vi "periodicTasksRefNum.vi"() -> (1 "Refnums":T28)   [LabVIEW 2016]
uses:
  <vilib>/Rock Robotics/WPI/RobotDrive/WPI_RobotDriveDevRef.ctl
  <vilib>/Rock Robotics/WPI/MotorControl/WPI_MotorControlDeviceRef.ctl
  <vilib>/Rock Robotics/WPI/MotorControl/WPI_MotorControlType.ctl
  <vilib>/Rock Robotics/SystemInterfaces/DIO/FPGA_DIOPWMChannel.ctl
  <vilib>/Rock Robotics/WPI/PWM/WPI_PWMDeadband.ctl
  Sensors/PixyCam/Private/PixyCam_DevRef.ctl
  Sensors/PixyCam/Private/PixyCam_SPI_DevRef.ctl
  <vilib>/Rock Robotics/WPI/SPI/WPI_SPIDevRef.ctl
  <vilib>/Rock Robotics/SystemInterfaces/spilib/spi_bus.ctl
  Sensors/PixyCam/Private/PixyCam_CommMode.ctl
  Sensors/ADI MXP IMU/ADI_IMU_ADIS16448_InterruptDevRef.ctl
  Sensors/ADI MXP IMU/ADI_IMU_ADIS16448_IMUDevRef.ctl
  <vilib>/Rock Robotics/WPI/Interrupt/WPI_InterruptRef.ctl
  <vilib>/Rock Robotics/SystemInterfaces/Interrupt/FPGA_InterruptIndex.ctl
  <vilib>/Rock Robotics/WPI/AnalogChannel/WPI_AnalogChannelDevRef.ctl
  <vilib>/Rock Robotics/SystemInterfaces/AI/FPGA_AIChannel.ctl
  <vilib>/Rock Robotics/WPI/Ultrasonic/WPI_SonarMB1010DigitalDeviceRef.ctl
  <vilib>/Rock Robotics/WPI/Counter/WPI_CounterDevRef.ctl
  <vilib>/Rock Robotics/SystemInterfaces/Counter/FPGA_CounterCtrSystemIndex.ctl
  <vilib>/Rock Robotics/WPI/Encoder/WPI_EncoderDevRef.ctl
  <vilib>/Rock Robotics/SystemInterfaces/Encoder/FPGA_EncoderIdx.ctl
  <vilib>/Rock Robotics/WPI/Encoder/WPI_EncoderType.ctl
  <vilib>/Rock Robotics/WPI/DigitalInput/WPI_DigitalInputDevRef.ctl
  <vilib>/Rock Robotics/SystemInterfaces/DIO/FPGA_DIOChannel.ctl
  <vilib>/Rock Robotics/WPI/Compressor/WPI_CompressorDevRef.ctl
  <vilib>/Rock Robotics/WPI/Solenoid/WPI_SolenoidDevRef.ctl
  <vilib>/Rock Robotics/WPI/Solenoid/WPI_SolenoidChannel.ctl
  <vilib>/Rock Robotics/WPI/Utilities/WPI_GetSetVariantRefNum.vi
  Sensors/ADI MXP IMU/ADIS16448_IMU.lvlib
  Sensors/PixyCam/PixyCam_LabVIEW.lvlib
types:
  T1 = typedef "WPI_RobotDriveDevRef.ctl" = cluster{"DevStatus":errorcluster, "Motors[]":T2[], "Square Inputs":bool, "Max Output":dbl}
  T2 = typedef "WPI_MotorControlDeviceRef.ctl" = cluster{"DeviceStatus":errorcluster, "Type":T3, "PWM":cluster{"PWM Channel":T4, "DeadBand":T5}, "CAN":cluster{"Device Number":u8, "SetOutput VI Ref":variant, "GetOutput VI Ref":variant, "Enable VI Ref":variant, "Disable VI Ref":variant, "Data":variant}, "Invert":bool}
  T3 = typedef "WPI_MotorControlType.ctl" = enum16{"PWM", "CAN"}
  T4 = typedef "FPGA_DIOPWMChannel.ctl" = enum8{"PWM 0", "PWM 1", "PWM 2", "PWM 3", "PWM 4", "PWM 5", "PWM 6", "PWM 7", "PWM 8", "PWM 9", "PWM MXP 0", "PWM MXP 1", "PWM MXP 2", "PWM MXP 3", "PWM MXP 4", "PWM MXP 5", "PWM MXP 6", "PWM MXP 7", "PWM MXP 8", "PWM MXP 9", "Invalid"}
  T5 = typedef "WPI_PWMDeadband.ctl" = cluster{"Name":string, "maxPositivePwm":i32, "minPositivePwm":i32, "centerPwm":i32, "maxNegativePwm":i32, "minNegativePwm":i32, "angularRange":u16}
  T6 = typedef "PixyCam_LabVIEW.lvlib/PixyCam_DevRef.ctl" = cluster{"PixyCamDevRef_SPI":T7, "Communication Mode":T10, "Error":errorcluster}
  T7 = typedef "PixyCam_LabVIEW.lvlib/PixyCam_SPI_DevRef.ctl" = cluster{"SPIDevRef":T8, "Output Queue":refnum<queue>}
  T8 = typedef "WPI_SPIDevRef.ctl" = cluster{"DevStatus":errorcluster, "Handle":i32, "SPI Bus":T9}
  T9 = typedef "spi_bus.ctl" = enum16{"SPI On-Board, CS0", "SPI On-Board, CS1", "SPI On-Board, CS2", "SPI On-Board, CS3", "SPI MXP", "Invalid"}
  T10 = typedef "PixyCam_LabVIEW.lvlib/PixyCam_CommMode.ctl" = enum16{"SPI", "I2C", "UART", "Analog", "Digital"}
  T11 = typedef "ADIS16448_IMU.lvlib/ADI_IMU_ADIS16448_InterruptDevRef.ctl" = cluster{"ADI IMU DevRef":T12, "InterruptRef":T13}
  T12 = typedef "ADIS16448_IMU.lvlib/ADI_IMU_ADIS16448_IMUDevRef.ctl" = cluster{"DevStatus":errorcluster, "Handle":i32, "SPI Bus":T9, "Device Found":bool, "Device Ready":bool, "Yaw Axis":enum16{"X", "Y", "Z"}, "AHRS Algorithm":enum16{"Complementary", "Madgwick"}, "Serial":u16, "Lot ID 2":u16, "Lot ID 1":u16, "Product ID":u16}
  T13 = typedef "WPI_InterruptRef.ctl" = cluster{"DevStatus":errorcluster, "InterruptIndex":T14}
  T14 = typedef "FPGA_InterruptIndex.ctl" = enum8{"0", "1", "2", "3", "4", "5", "6", "7", "Invalid"}
  T15 = typedef "WPI_AnalogChannelDevRef.ctl" = cluster{"DevStatus":errorcluster, "Analog Channel":T16}
  T16 = typedef "FPGA_AIChannel.ctl" = enum8{"AI 0", "AI 1", "AI 2", "AI 3", "AI MXP 0", "AI MXP 1", "AI MXP 2", "AI MXP 3", "Invalid"}
  T17 = typedef "WPI_SonarMB1010DigitalDeviceRef.ctl" = cluster{"CounterDevRef":T18, "Scaling factor (s/in)":dbl}
  T18 = typedef "WPI_CounterDevRef.ctl" = cluster{"DevStatus":errorcluster, "CntIndex":T19}
  T19 = typedef "FPGA_CounterCtrSystemIndex.ctl" = enum8{"Ctr 0", "Ctr 1", "Ctr 2", "Ctr 3", "Ctr 4", "Ctr 5", "Ctr 6", "Ctr 7", "Invalid"}
  T20 = typedef "WPI_EncoderDevRef.ctl" = cluster{"DevStatus":errorcluster, "EncoderIndex":T21, "CounterIndex":T19, "DistancePerCount":dbl, "Decoding Type":T22}
  T21 = typedef "FPGA_EncoderIdx.ctl" = enum8{"Enc 0", "Enc 1", "Enc 2", "Enc 3", "Enc 4", "Enc 5", "Enc 6", "Enc 7", "Invalid"}
  T22 = typedef "WPI_EncoderType.ctl" = enum16{"1x", "2x", "4x"}
  T23 = typedef "WPI_DigitalInputDevRef.ctl" = cluster{"DevStatus":errorcluster, "DIO Channel":T24}
  T24 = typedef "FPGA_DIOChannel.ctl" = enum8{"DIO 0", "DIO 1", "DIO 2", "DIO 3", "DIO 4", "DIO 5", "DIO 6", "DIO 7", "DIO 8", "DIO 9", "DIO MXP 0", "DIO MXP 1", "DIO MXP 2", "DIO MXP 3", "DIO MXP 4", "DIO MXP 5", "DIO MXP 6", "DIO MXP 7", "DIO MXP 8", "DIO MXP 9", "DIO MXP 10", "DIO MXP 11", "DIO MXP 12", "DIO MXP 13", "DIO MXP 14", "DIO MXP 15", "SPI Port CS1", "SPI Port CS2", "SPI Port CS3", "SPI Port MISO", "SPI Port MOSI", "Invalid"}
  T25 = typedef "WPI_CompressorDevRef.ctl" = cluster{"DevStatus":errorcluster, "Pneumatics Control Module":u8}
  T26 = typedef "WPI_SolenoidDevRef.ctl" = cluster{"DevStatus":errorcluster, "Pneumatics Control Module":u8, "Forward Solenoid Channel":T27, "Reverse Solenoid Channel":T27}
  T27 = typedef "WPI_SolenoidChannel.ctl" = enum8{"Solenoid 0", "Solenoid 1", "Solenoid 2", "Solenoid 3", "Solenoid 4", "Solenoid 5", "Solenoid 6", "Solenoid 7", "Invalid"}
  T28 = cluster{"Motors":cluster{"Drive_Motor":cluster{"RobotDriveDevRef":T1, "error out":errorcluster}, "Shooter_Motor":cluster{"MotorControlDevRef":T2, "error out":errorcluster}, "Shooter_Feeder_Motor":cluster{"MotorControlDevRef":T2, "error out":errorcluster}, "Intake_Motor_1":cluster{"MotorControlDevRef":T2, "error out":errorcluster}, "Gear_Gate_Motor":cluster{"MotorControlDevRef":T2, "error out":errorcluster}, "Climber_Motor":cluster{"MotorControlDevRef":T2, "error out":errorcluster}, "Shooter_Turret_Motor":cluster{"MotorControlDevRef":T2, "error out":errorcluster}, "Top_Shooter_Feeder_Motor":cluster{"MotorControlDevRef":T2, "error out":errorcluster}, "Gear_Rail_Motor":cluster{"MotorControlDevRef":T2, "error out":errorcluster}}, "Sensors":cluster{"PixyCam":cluster{"PixyCamDevRef Out":T6, "error out":errorcluster}, "IMU":cluster{"ADI IMU Interrupt DevRef":T11, "error out":errorcluster}, "Pots":cluster{"Gear_Gate_Pot":cluster{"AIDeviceRef":T15, "error out":errorcluster}, "Gear_Rail_Pot":cluster{"AIDeviceRef":T15, "error out":errorcluster}, "Turret_Pot":cluster{"AIDeviceRef":T15, "error out":errorcluster}}, "Ultrasonics":cluster{"Gear_Peg_Ultrasonic":cluster{"SonarMB1010DigitalDevRef":T17, "error out":errorcluster}}, "Encoders":cluster{"Drive_Encoder":cluster{"EncoderDevRef":T20, "error out":errorcluster}, "Shooter_Encoder":cluster{"EncoderDevRef":T20, "error out":errorcluster}}, "DIOs":cluster{"Gear_Beambreak":cluster{"DigitalInputDevRef":T23, "error out":errorcluster}, "Ball_Beambreak":cluster{"DigitalInputDevRef":T23, "error out":errorcluster}, "Gear_Orientation_Beambreak":cluster{"DigitalInputDevRef":T23, "error out":errorcluster}}}, "Pneumatics":cluster{"Compressor":cluster{"CompressorDevRef":T25, "error out":errorcluster}, "Gear_Pusher":cluster{"SolenoidDevRef":T26, "error out":errorcluster}, "Shifters":cluster{"SolenoidDevRef":T26, "error out":errorcluster}, "Gear_Chute":cluster{"SolenoidDevRef":T26, "error out":errorcluster}}}
  T29 = cluster{"PixyCam":cluster{"PixyCamDevRef Out":T6, "error out":errorcluster}, "IMU":cluster{"ADI IMU Interrupt DevRef":T11, "error out":errorcluster}, "Pots":cluster{"Gear_Gate_Pot":cluster{"AIDeviceRef":T15, "error out":errorcluster}, "Gear_Rail_Pot":cluster{"AIDeviceRef":T15, "error out":errorcluster}, "Turret_Pot":cluster{"AIDeviceRef":T15, "error out":errorcluster}}, "Ultrasonics":cluster{"Gear_Peg_Ultrasonic":cluster{"SonarMB1010DigitalDevRef":T17, "error out":errorcluster}}, "Encoders":cluster{"Drive_Encoder":cluster{"EncoderDevRef":T20, "error out":errorcluster}, "Shooter_Encoder":cluster{"EncoderDevRef":T20, "error out":errorcluster}}, "DIOs":cluster{"Gear_Beambreak":cluster{"DigitalInputDevRef":T23, "error out":errorcluster}, "Ball_Beambreak":cluster{"DigitalInputDevRef":T23, "error out":errorcluster}, "Gear_Orientation_Beambreak":cluster{"DigitalInputDevRef":T23, "error out":errorcluster}}}
  T30 = cluster{"Gear_Beambreak":cluster{"DigitalInputDevRef":T23, "error out":errorcluster}, "Ball_Beambreak":cluster{"DigitalInputDevRef":T23, "error out":errorcluster}, "Gear_Orientation_Beambreak":cluster{"DigitalInputDevRef":T23, "error out":errorcluster}}
  T31 = cluster{"DigitalInputDevRef":T23, "error out":errorcluster}
  T32 = cluster{"Gear_Peg_Ultrasonic":cluster{"SonarMB1010DigitalDevRef":T17, "error out":errorcluster}}
  T33 = cluster{"SonarMB1010DigitalDevRef":T17, "error out":errorcluster}
  T34 = cluster{"PixyCamDevRef Out":T6, "error out":errorcluster}
  T35 = cluster{"Drive_Motor":cluster{"RobotDriveDevRef":T1, "error out":errorcluster}, "Shooter_Motor":cluster{"MotorControlDevRef":T2, "error out":errorcluster}, "Shooter_Feeder_Motor":cluster{"MotorControlDevRef":T2, "error out":errorcluster}, "Intake_Motor_1":cluster{"MotorControlDevRef":T2, "error out":errorcluster}, "Gear_Gate_Motor":cluster{"MotorControlDevRef":T2, "error out":errorcluster}, "Climber_Motor":cluster{"MotorControlDevRef":T2, "error out":errorcluster}, "Shooter_Turret_Motor":cluster{"MotorControlDevRef":T2, "error out":errorcluster}, "Top_Shooter_Feeder_Motor":cluster{"MotorControlDevRef":T2, "error out":errorcluster}, "Gear_Rail_Motor":cluster{"MotorControlDevRef":T2, "error out":errorcluster}}
  T36 = cluster{"MotorControlDevRef":T2, "error out":errorcluster}
  T37 = cluster{"Gear_Gate_Pot":cluster{"AIDeviceRef":T15, "error out":errorcluster}, "Gear_Rail_Pot":cluster{"AIDeviceRef":T15, "error out":errorcluster}, "Turret_Pot":cluster{"AIDeviceRef":T15, "error out":errorcluster}}
  T38 = cluster{"AIDeviceRef":T15, "error out":errorcluster}
  T39 = cluster{"Compressor":cluster{"CompressorDevRef":T25, "error out":errorcluster}, "Gear_Pusher":cluster{"SolenoidDevRef":T26, "error out":errorcluster}, "Shifters":cluster{"SolenoidDevRef":T26, "error out":errorcluster}, "Gear_Chute":cluster{"SolenoidDevRef":T26, "error out":errorcluster}}
  T40 = cluster{"SolenoidDevRef":T26, "error out":errorcluster}
  T41 = cluster{"Drive_Encoder":cluster{"EncoderDevRef":T20, "error out":errorcluster}, "Shooter_Encoder":cluster{"EncoderDevRef":T20, "error out":errorcluster}}
  T42 = cluster{"EncoderDevRef":T20, "error out":errorcluster}
  T43 = cluster{"ADI IMU Interrupt DevRef":T11, "error out":errorcluster}
  T44 = cluster{"CompressorDevRef":T25, "error out":errorcluster}
  T45 = cluster{"RobotDriveDevRef":T1, "error out":errorcluster}
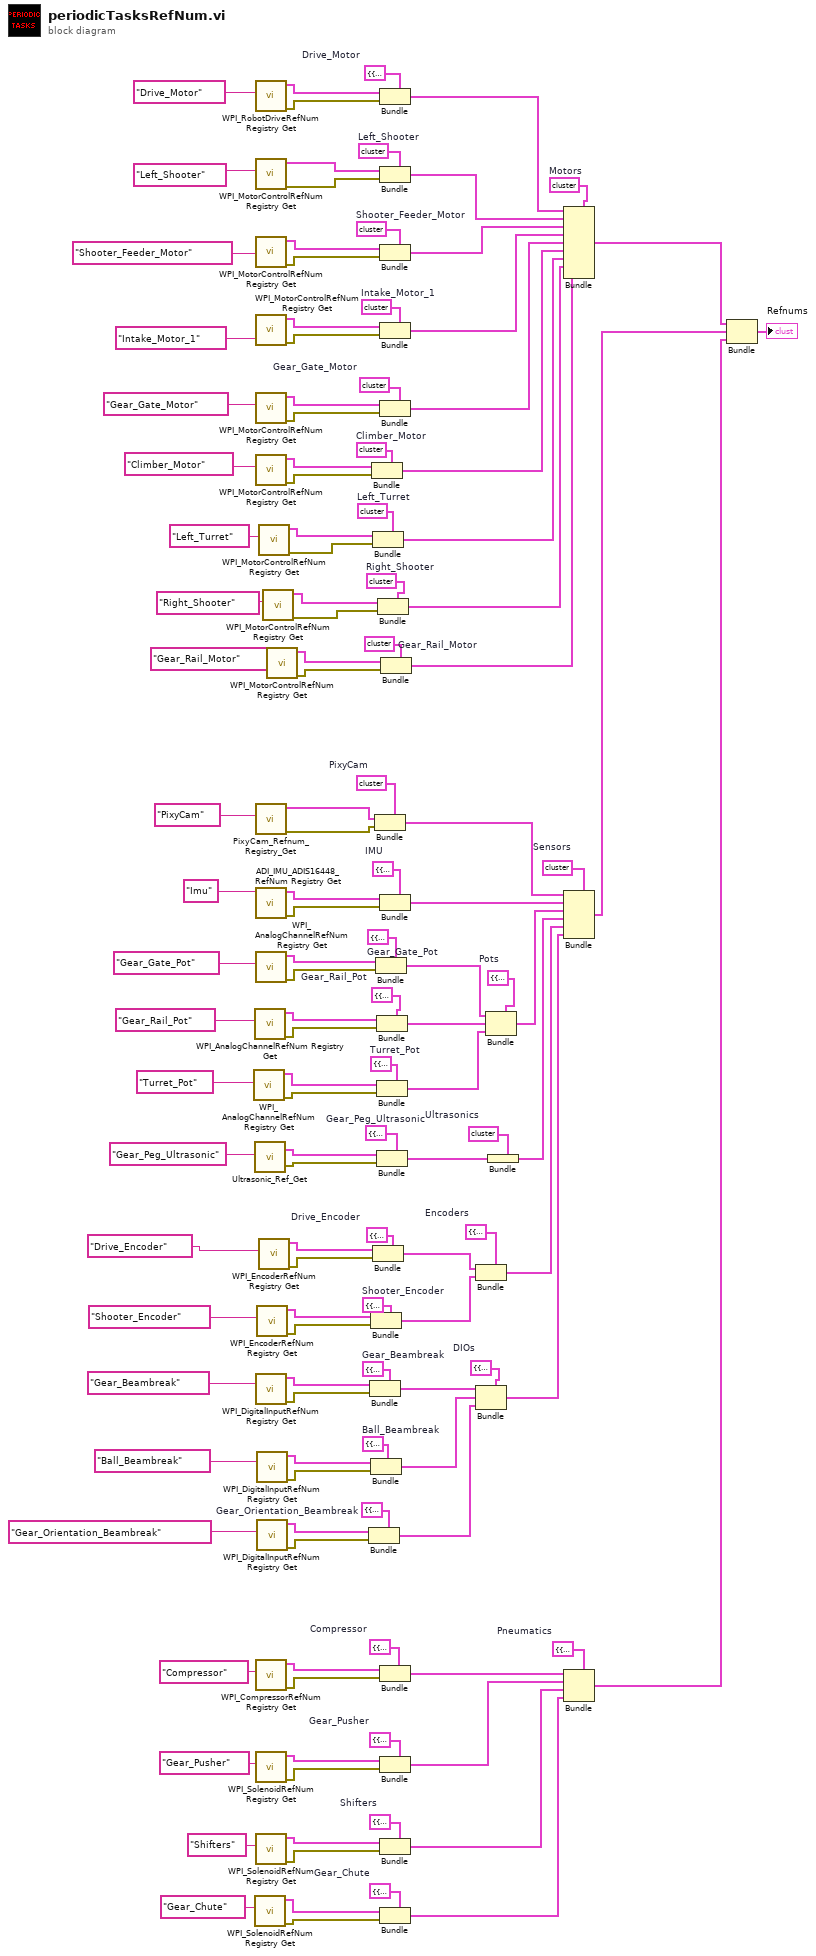
[diagram p0: block diagram]
diagram:
  w2 = T29 {"PixyCam"={"PixyCamDevRef Out"={"PixyCamDevRef_SPI"={"SPIDevRef"={"DevStatus"={"status"=FALSE, "code"=0, "source"=""}, "Handle"=0, "SPI Bus"=enum."SPI On-Board, CS0"}, "Output Queue"=refnum}, "Communication Mode"=enum."SPI", "Error"={"status"=FALSE, "code"=0, "source"=""}}, "error out"={"status"=FALSE, "code"=0, "source"=""}}, "IMU"={"ADI IMU Interrupt DevRef"={"ADI IMU DevRef"={"DevStatus"={"status"=FALSE, "code"=0, "source"=""}, "Handle"=0, "SPI Bus"=enum."SPI On-Board, CS0", "Device Found"=FALSE, "Device Ready"=FALSE, "Yaw Axis"=enum."X", "AHRS Algorithm"=enum."Complementary", "Serial"=0, "Lot ID 2"=0, "Lot ID 1"=0, "Product ID"=0}, "InterruptRef"={"DevStatus"={"status"=FALSE, "code"=0, "source"=""}, "InterruptIndex"=enum."0"}}, "error out"={"status"=FALSE, "code"=0, "source"=""}}, "Pots"={"Gear_Gate_Pot"={"AIDeviceRef"={"DevStatus"={"status"=FALSE, "code"=0, "source"=""}, "Analog Channel"=enum."AI 0"}, "error out"={"status"=FALSE, "code"=0, "source"=""}}, "Gear_Rail_Pot"={"AIDeviceRef"={"DevStatus"={"status"=FALSE, "code"=0, "source"=""}, "Analog Channel"=enum."AI 0"}, "error out"={"status"=FALSE, "code"=0, "source"=""}}, "Turret_Pot"={"AIDeviceRef"={"DevStatus"={"status"=FALSE, "code"=0, "source"=""}, "Analog Channel"=enum."AI 0"}, "error out"={"status"=FALSE, "code"=0, "source"=""}}}, "Ultrasonics"={"Gear_Peg_Ultrasonic"={"SonarMB1010DigitalDevRef"={"CounterDevRef"={"DevStatus"={"status"=FALSE, "code"=0, "source"=""}, "CntIndex"=enum."Ctr 0"}, "Scaling factor (s/in)"=0.0}, "error out"={"status"=FALSE, "code"=0, "source"=""}}}, "Encoders"={"Drive_Encoder"={"EncoderDevRef"={"DevStatus"={"status"=FALSE, "code"=0, "source"=""}, "EncoderIndex"=enum."Enc 0", "CounterIndex"=enum."Ctr 0", "DistancePerCount"=0.0, "Decoding Type"=enum."1x"}, "error out"={"status"=FALSE, "code"=0, "source"=""}}, "Shooter_Encoder"={"EncoderDevRef"={"DevStatus"={"status"=FALSE, "code"=0, "source"=""}, "EncoderIndex"=enum."Enc 0", "CounterIndex"=enum."Ctr 0", "DistancePerCount"=0.0, "Decoding Type"=enum."1x"}, "error out"={"status"=FALSE, "code"=0, "source"=""}}}, "DIOs"={"Gear_Beambreak"={"DigitalInputDevRef"={"DevStatus"={"status"=FALSE, "code"=0, "source"=""}, "DIO Channel"=enum."DIO 0"}, "error out"={"status"=FALSE, "code"=0, "source"=""}}, "Ball_Beambreak"={"DigitalInputDevRef"={"DevStatus"={"status"=FALSE, "code"=0, "source"=""}, "DIO Channel"=enum."DIO 0"}, "error out"={"status"=FALSE, "code"=0, "source"=""}}, "Gear_Orientation_Beambreak"={"DigitalInputDevRef"={"DevStatus"={"status"=FALSE, "code"=0, "source"=""}, "DIO Channel"=enum."DIO 0"}, "error out"={"status"=FALSE, "code"=0, "source"=""}}}}  # Sensors
  w3 = T30 {"Gear_Beambreak"={"DigitalInputDevRef"={"DevStatus"={"status"=FALSE, "code"=0, "source"=""}, "DIO Channel"=enum."DIO 0"}, "error out"={"status"=FALSE, "code"=0, "source"=""}}, "Ball_Beambreak"={"DigitalInputDevRef"={"DevStatus"={"status"=FALSE, "code"=0, "source"=""}, "DIO Channel"=enum."DIO 0"}, "error out"={"status"=FALSE, "code"=0, "source"=""}}, "Gear_Orientation_Beambreak"={"DigitalInputDevRef"={"DevStatus"={"status"=FALSE, "code"=0, "source"=""}, "DIO Channel"=enum."DIO 0"}, "error out"={"status"=FALSE, "code"=0, "source"=""}}}  # DIOs
  w4 = T31 {"DigitalInputDevRef"={"DevStatus"={"status"=FALSE, "code"=0, "source"=""}, "DIO Channel"=enum."DIO 0"}, "error out"={"status"=FALSE, "code"=0, "source"=""}}  # Gear_Orientation_Beambreak
  w9 = T32 {"Gear_Peg_Ultrasonic"={"SonarMB1010DigitalDevRef"={"CounterDevRef"={"DevStatus"={"status"=FALSE, "code"=0, "source"=""}, "CntIndex"=enum."Ctr 0"}, "Scaling factor (s/in)"=0.0}, "error out"={"status"=FALSE, "code"=0, "source"=""}}}  # Ultrasonics
  w10 = T33 {"SonarMB1010DigitalDevRef"={"CounterDevRef"={"DevStatus"={"status"=FALSE, "code"=0, "source"=""}, "CntIndex"=enum."Ctr 0"}, "Scaling factor (s/in)"=0.0}, "error out"={"status"=FALSE, "code"=0, "source"=""}}  # Gear_Peg_Ultrasonic
  w12 = T34 {"PixyCamDevRef Out"={"PixyCamDevRef_SPI"={"SPIDevRef"={"DevStatus"={"status"=FALSE, "code"=0, "source"=""}, "Handle"=0, "SPI Bus"=enum."SPI On-Board, CS0"}, "Output Queue"=refnum}, "Communication Mode"=enum."SPI", "Error"={"status"=FALSE, "code"=0, "source"=""}}, "error out"={"status"=FALSE, "code"=0, "source"=""}}  # PixyCam
  w16 = T35 {"Drive_Motor"={"RobotDriveDevRef"={"DevStatus"={"status"=FALSE, "code"=0, "source"=""}, "Motors[]"=[], "Square Inputs"=FALSE, "Max Output"=0.0}, "error out"={"status"=FALSE, "code"=0, "source"=""}}, "Shooter_Motor"={"MotorControlDevRef"={"DeviceStatus"={"status"=FALSE, "code"=0, "source"=""}, "Type"=enum."PWM", "PWM"={"PWM Channel"=enum."PWM 0", "DeadBand"={"Name"="", "maxPositivePwm"=0, "minPositivePwm"=0, "centerPwm"=0, "maxNegativePwm"=0, "minNegativePwm"=0, "angularRange"=0}}, "CAN"={"Device Number"=0, "SetOutput VI Ref"=variant, "GetOutput VI Ref"=variant, "Enable VI Ref"=variant, "Disable VI Ref"=variant, "Data"=variant}, "Invert"=FALSE}, "error out"={"status"=FALSE, "code"=0, "source"=""}}, "Shooter_Feeder_Motor"={"MotorControlDevRef"={"DeviceStatus"={"status"=FALSE, "code"=0, "source"=""}, "Type"=enum."PWM", "PWM"={"PWM Channel"=enum."PWM 0", "DeadBand"={"Name"="", "maxPositivePwm"=0, "minPositivePwm"=0, "centerPwm"=0, "maxNegativePwm"=0, "minNegativePwm"=0, "angularRange"=0}}, "CAN"={"Device Number"=0, "SetOutput VI Ref"=variant, "GetOutput VI Ref"=variant, "Enable VI Ref"=variant, "Disable VI Ref"=variant, "Data"=variant}, "Invert"=FALSE}, "error out"={"status"=FALSE, "code"=0, "source"=""}}, "Intake_Motor_1"={"MotorControlDevRef"={"DeviceStatus"={"status"=FALSE, "code"=0, "source"=""}, "Type"=enum."PWM", "PWM"={"PWM Channel"=enum."PWM 0", "DeadBand"={"Name"="", "maxPositivePwm"=0, "minPositivePwm"=0, "centerPwm"=0, "maxNegativePwm"=0, "minNegativePwm"=0, "angularRange"=0}}, "CAN"={"Device Number"=0, "SetOutput VI Ref"=variant, "GetOutput VI Ref"=variant, "Enable VI Ref"=variant, "Disable VI Ref"=variant, "Data"=variant}, "Invert"=FALSE}, "error out"={"status"=FALSE, "code"=0, "source"=""}}, "Gear_Gate_Motor"={"MotorControlDevRef"={"DeviceStatus"={"status"=FALSE, "code"=0, "source"=""}, "Type"=enum."PWM", "PWM"={"PWM Channel"=enum."PWM 0", "DeadBand"={"Name"="", "maxPositivePwm"=0, "minPositivePwm"=0, "centerPwm"=0, "maxNegativePwm"=0, "minNegativePwm"=0, "angularRange"=0}}, "CAN"={"Device Number"=0, "SetOutput VI Ref"=variant, "GetOutput VI Ref"=variant, "Enable VI Ref"=variant, "Disable VI Ref"=variant, "Data"=variant}, "Invert"=FALSE}, "error out"={"status"=FALSE, "code"=0, "source"=""}}, "Climber_Motor"={"MotorControlDevRef"={"DeviceStatus"={"status"=FALSE, "code"=0, "source"=""}, "Type"=enum."PWM", "PWM"={"PWM Channel"=enum."PWM 0", "DeadBand"={"Name"="", "maxPositivePwm"=0, "minPositivePwm"=0, "centerPwm"=0, "maxNegativePwm"=0, "minNegativePwm"=0, "angularRange"=0}}, "CAN"={"Device Number"=0, "SetOutput VI Ref"=variant, "GetOutput VI Ref"=variant, "Enable VI Ref"=variant, "Disable VI Ref"=variant, "Data"=variant}, "Invert"=FALSE}, "error out"={"status"=FALSE, "code"=0, "source"=""}}, "Shooter_Turret_Motor"={"MotorControlDevRef"={"DeviceStatus"={"status"=FALSE, "code"=0, "source"=""}, "Type"=enum."PWM", "PWM"={"PWM Channel"=enum."PWM 0", "DeadBand"={"Name"="", "maxPositivePwm"=0, "minPositivePwm"=0, "centerPwm"=0, "maxNegativePwm"=0, "minNegativePwm"=0, "angularRange"=0}}, "CAN"={"Device Number"=0, "SetOutput VI Ref"=variant, "GetOutput VI Ref"=variant, "Enable VI Ref"=variant, "Disable VI Ref"=variant, "Data"=variant}, "Invert"=FALSE}, "error out"={"status"=FALSE, "code"=0, "source"=""}}, "Top_Shooter_Feeder_Motor"={"MotorControlDevRef"={"DeviceStatus"={"status"=FALSE, "code"=0, "source"=""}, "Type"=enum."PWM", "PWM"={"PWM Channel"=enum."PWM 0", "DeadBand"={"Name"="", "maxPositivePwm"=0, "minPositivePwm"=0, "centerPwm"=0, "maxNegativePwm"=0, "minNegativePwm"=0, "angularRange"=0}}, "CAN"={"Device Number"=0, "SetOutput VI Ref"=variant, "GetOutput VI Ref"=variant, "Enable VI Ref"=variant, "Disable VI Ref"=variant, "Data"=variant}, "Invert"=FALSE}, "error out"={"status"=FALSE, "code"=0, "source"=""}}, "Gear_Rail_Motor"={"MotorControlDevRef"={"DeviceStatus"={"status"=FALSE, "code"=0, "source"=""}, "Type"=enum."PWM", "PWM"={"PWM Channel"=enum."PWM 0", "DeadBand"={"Name"="", "maxPositivePwm"=0, "minPositivePwm"=0, "centerPwm"=0, "maxNegativePwm"=0, "minNegativePwm"=0, "angularRange"=0}}, "CAN"={"Device Number"=0, "SetOutput VI Ref"=variant, "GetOutput VI Ref"=variant, "Enable VI Ref"=variant, "Disable VI Ref"=variant, "Data"=variant}, "Invert"=FALSE}, "error out"={"status"=FALSE, "code"=0, "source"=""}}}  # Motors
  w17 = T36 {"MotorControlDevRef"={"DeviceStatus"={"status"=FALSE, "code"=0, "source"=""}, "Type"=enum."PWM", "PWM"={"PWM Channel"=enum."PWM 0", "DeadBand"={"Name"="", "maxPositivePwm"=0, "minPositivePwm"=0, "centerPwm"=0, "maxNegativePwm"=0, "minNegativePwm"=0, "angularRange"=0}}, "CAN"={"Device Number"=0, "SetOutput VI Ref"=variant, "GetOutput VI Ref"=variant, "Enable VI Ref"=variant, "Disable VI Ref"=variant, "Data"=variant}, "Invert"=FALSE}, "error out"={"status"=FALSE, "code"=0, "source"=""}}  # Gear_Rail_Motor
  w22 = T37 {"Gear_Gate_Pot"={"AIDeviceRef"={"DevStatus"={"status"=FALSE, "code"=0, "source"=""}, "Analog Channel"=enum."AI 0"}, "error out"={"status"=FALSE, "code"=0, "source"=""}}, "Gear_Rail_Pot"={"AIDeviceRef"={"DevStatus"={"status"=FALSE, "code"=0, "source"=""}, "Analog Channel"=enum."AI 0"}, "error out"={"status"=FALSE, "code"=0, "source"=""}}, "Turret_Pot"={"AIDeviceRef"={"DevStatus"={"status"=FALSE, "code"=0, "source"=""}, "Analog Channel"=enum."AI 0"}, "error out"={"status"=FALSE, "code"=0, "source"=""}}}  # Pots
  w23 = T38 {"AIDeviceRef"={"DevStatus"={"status"=FALSE, "code"=0, "source"=""}, "Analog Channel"=enum."AI 0"}, "error out"={"status"=FALSE, "code"=0, "source"=""}}  # Gear_Gate_Pot
  w24 = T38 {"AIDeviceRef"={"DevStatus"={"status"=FALSE, "code"=0, "source"=""}, "Analog Channel"=enum."AI 0"}, "error out"={"status"=FALSE, "code"=0, "source"=""}}  # Gear_Rail_Pot
  w25 = T38 {"AIDeviceRef"={"DevStatus"={"status"=FALSE, "code"=0, "source"=""}, "Analog Channel"=enum."AI 0"}, "error out"={"status"=FALSE, "code"=0, "source"=""}}  # Turret_Pot
  w30 = T36 {"MotorControlDevRef"={"DeviceStatus"={"status"=FALSE, "code"=0, "source"=""}, "Type"=enum."PWM", "PWM"={"PWM Channel"=enum."PWM 0", "DeadBand"={"Name"="", "maxPositivePwm"=0, "minPositivePwm"=0, "centerPwm"=0, "maxNegativePwm"=0, "minNegativePwm"=0, "angularRange"=0}}, "CAN"={"Device Number"=0, "SetOutput VI Ref"=variant, "GetOutput VI Ref"=variant, "Enable VI Ref"=variant, "Disable VI Ref"=variant, "Data"=variant}, "Invert"=FALSE}, "error out"={"status"=FALSE, "code"=0, "source"=""}}  # Right_Shooter
  w38 = T31 {"DigitalInputDevRef"={"DevStatus"={"status"=FALSE, "code"=0, "source"=""}, "DIO Channel"=enum."DIO 0"}, "error out"={"status"=FALSE, "code"=0, "source"=""}}  # Ball_Beambreak
  w39 = T39 {"Compressor"={"CompressorDevRef"={"DevStatus"={"status"=FALSE, "code"=0, "source"=""}, "Pneumatics Control Module"=0}, "error out"={"status"=FALSE, "code"=0, "source"=""}}, "Gear_Pusher"={"SolenoidDevRef"={"DevStatus"={"status"=FALSE, "code"=0, "source"=""}, "Pneumatics Control Module"=0, "Forward Solenoid Channel"=enum."Solenoid 0", "Reverse Solenoid Channel"=enum."Solenoid 0"}, "error out"={"status"=FALSE, "code"=0, "source"=""}}, "Shifters"={"SolenoidDevRef"={"DevStatus"={"status"=FALSE, "code"=0, "source"=""}, "Pneumatics Control Module"=0, "Forward Solenoid Channel"=enum."Solenoid 0", "Reverse Solenoid Channel"=enum."Solenoid 0"}, "error out"={"status"=FALSE, "code"=0, "source"=""}}, "Gear_Chute"={"SolenoidDevRef"={"DevStatus"={"status"=FALSE, "code"=0, "source"=""}, "Pneumatics Control Module"=0, "Forward Solenoid Channel"=enum."Solenoid 0", "Reverse Solenoid Channel"=enum."Solenoid 0"}, "error out"={"status"=FALSE, "code"=0, "source"=""}}}  # Pneumatics
  w41 = T40 {"SolenoidDevRef"={"DevStatus"={"status"=FALSE, "code"=0, "source"=""}, "Pneumatics Control Module"=0, "Forward Solenoid Channel"=enum."Solenoid 0", "Reverse Solenoid Channel"=enum."Solenoid 0"}, "error out"={"status"=FALSE, "code"=0, "source"=""}}  # Gear_Chute
  w53 = T41 {"Drive_Encoder"={"EncoderDevRef"={"DevStatus"={"status"=FALSE, "code"=0, "source"=""}, "EncoderIndex"=enum."Enc 0", "CounterIndex"=enum."Ctr 0", "DistancePerCount"=0.0, "Decoding Type"=enum."1x"}, "error out"={"status"=FALSE, "code"=0, "source"=""}}, "Shooter_Encoder"={"EncoderDevRef"={"DevStatus"={"status"=FALSE, "code"=0, "source"=""}, "EncoderIndex"=enum."Enc 0", "CounterIndex"=enum."Ctr 0", "DistancePerCount"=0.0, "Decoding Type"=enum."1x"}, "error out"={"status"=FALSE, "code"=0, "source"=""}}}  # Encoders
  w54 = T31 {"DigitalInputDevRef"={"DevStatus"={"status"=FALSE, "code"=0, "source"=""}, "DIO Channel"=enum."DIO 0"}, "error out"={"status"=FALSE, "code"=0, "source"=""}}  # Gear_Beambreak
  w55 = T42 {"EncoderDevRef"={"DevStatus"={"status"=FALSE, "code"=0, "source"=""}, "EncoderIndex"=enum."Enc 0", "CounterIndex"=enum."Ctr 0", "DistancePerCount"=0.0, "Decoding Type"=enum."1x"}, "error out"={"status"=FALSE, "code"=0, "source"=""}}  # Shooter_Encoder
  w56 = T42 {"EncoderDevRef"={"DevStatus"={"status"=FALSE, "code"=0, "source"=""}, "EncoderIndex"=enum."Enc 0", "CounterIndex"=enum."Ctr 0", "DistancePerCount"=0.0, "Decoding Type"=enum."1x"}, "error out"={"status"=FALSE, "code"=0, "source"=""}}  # Drive_Encoder
  w78 = T36 {"MotorControlDevRef"={"DeviceStatus"={"status"=FALSE, "code"=0, "source"=""}, "Type"=enum."PWM", "PWM"={"PWM Channel"=enum."PWM 0", "DeadBand"={"Name"="", "maxPositivePwm"=0, "minPositivePwm"=0, "centerPwm"=0, "maxNegativePwm"=0, "minNegativePwm"=0, "angularRange"=0}}, "CAN"={"Device Number"=0, "SetOutput VI Ref"=variant, "GetOutput VI Ref"=variant, "Enable VI Ref"=variant, "Disable VI Ref"=variant, "Data"=variant}, "Invert"=FALSE}, "error out"={"status"=FALSE, "code"=0, "source"=""}}  # Left_Turret
  w84 = T36 {"MotorControlDevRef"={"DeviceStatus"={"status"=FALSE, "code"=0, "source"=""}, "Type"=enum."PWM", "PWM"={"PWM Channel"=enum."PWM 0", "DeadBand"={"Name"="", "maxPositivePwm"=0, "minPositivePwm"=0, "centerPwm"=0, "maxNegativePwm"=0, "minNegativePwm"=0, "angularRange"=0}}, "CAN"={"Device Number"=0, "SetOutput VI Ref"=variant, "GetOutput VI Ref"=variant, "Enable VI Ref"=variant, "Disable VI Ref"=variant, "Data"=variant}, "Invert"=FALSE}, "error out"={"status"=FALSE, "code"=0, "source"=""}}  # Climber_Motor
  w88 = T43 {"ADI IMU Interrupt DevRef"={"ADI IMU DevRef"={"DevStatus"={"status"=FALSE, "code"=0, "source"=""}, "Handle"=0, "SPI Bus"=enum."SPI On-Board, CS0", "Device Found"=FALSE, "Device Ready"=FALSE, "Yaw Axis"=enum."X", "AHRS Algorithm"=enum."Complementary", "Serial"=0, "Lot ID 2"=0, "Lot ID 1"=0, "Product ID"=0}, "InterruptRef"={"DevStatus"={"status"=FALSE, "code"=0, "source"=""}, "InterruptIndex"=enum."0"}}, "error out"={"status"=FALSE, "code"=0, "source"=""}}  # IMU
  w93 = T40 {"SolenoidDevRef"={"DevStatus"={"status"=FALSE, "code"=0, "source"=""}, "Pneumatics Control Module"=0, "Forward Solenoid Channel"=enum."Solenoid 0", "Reverse Solenoid Channel"=enum."Solenoid 0"}, "error out"={"status"=FALSE, "code"=0, "source"=""}}  # Gear_Pusher
  w95 = T40 {"SolenoidDevRef"={"DevStatus"={"status"=FALSE, "code"=0, "source"=""}, "Pneumatics Control Module"=0, "Forward Solenoid Channel"=enum."Solenoid 0", "Reverse Solenoid Channel"=enum."Solenoid 0"}, "error out"={"status"=FALSE, "code"=0, "source"=""}}  # Shifters
  w100 = T36 {"MotorControlDevRef"={"DeviceStatus"={"status"=FALSE, "code"=0, "source"=""}, "Type"=enum."PWM", "PWM"={"PWM Channel"=enum."PWM 0", "DeadBand"={"Name"="", "maxPositivePwm"=0, "minPositivePwm"=0, "centerPwm"=0, "maxNegativePwm"=0, "minNegativePwm"=0, "angularRange"=0}}, "CAN"={"Device Number"=0, "SetOutput VI Ref"=variant, "GetOutput VI Ref"=variant, "Enable VI Ref"=variant, "Disable VI Ref"=variant, "Data"=variant}, "Invert"=FALSE}, "error out"={"status"=FALSE, "code"=0, "source"=""}}  # Gear_Gate_Motor
  w106 = T44 {"CompressorDevRef"={"DevStatus"={"status"=FALSE, "code"=0, "source"=""}, "Pneumatics Control Module"=0}, "error out"={"status"=FALSE, "code"=0, "source"=""}}  # Compressor
  w117 = T36 {"MotorControlDevRef"={"DeviceStatus"={"status"=FALSE, "code"=0, "source"=""}, "Type"=enum."PWM", "PWM"={"PWM Channel"=enum."PWM 0", "DeadBand"={"Name"="", "maxPositivePwm"=0, "minPositivePwm"=0, "centerPwm"=0, "maxNegativePwm"=0, "minNegativePwm"=0, "angularRange"=0}}, "CAN"={"Device Number"=0, "SetOutput VI Ref"=variant, "GetOutput VI Ref"=variant, "Enable VI Ref"=variant, "Disable VI Ref"=variant, "Data"=variant}, "Invert"=FALSE}, "error out"={"status"=FALSE, "code"=0, "source"=""}}  # Intake_Motor_1
  w127 = T36 {"MotorControlDevRef"={"DeviceStatus"={"status"=FALSE, "code"=0, "source"=""}, "Type"=enum."PWM", "PWM"={"PWM Channel"=enum."PWM 0", "DeadBand"={"Name"="", "maxPositivePwm"=0, "minPositivePwm"=0, "centerPwm"=0, "maxNegativePwm"=0, "minNegativePwm"=0, "angularRange"=0}}, "CAN"={"Device Number"=0, "SetOutput VI Ref"=variant(enum8{"Percent VBus", "Current", "Speed", "Position", "Voltage"} enum."Percent VBus"), "GetOutput VI Ref"=variant(refnum<k1> refnum), "Enable VI Ref"=variant(dbl 0.0), "Disable VI Ref"=variant(enum8{"Percent VBus", "Speed", "Position", "Slave", "Unchanged / Invalid", "Voltage Compensation", "Current", "Motion Profile"} enum."Percent VBus"), "Data"=variant}, "Invert"=FALSE}, "error out"={"status"=FALSE, "code"=0, "source"=""}}  # Shooter_Feeder_Motor
  w128 = T36 {"MotorControlDevRef"={"DeviceStatus"={"status"=FALSE, "code"=0, "source"=""}, "Type"=enum."PWM", "PWM"={"PWM Channel"=enum."PWM 0", "DeadBand"={"Name"="", "maxPositivePwm"=0, "minPositivePwm"=0, "centerPwm"=0, "maxNegativePwm"=0, "minNegativePwm"=0, "angularRange"=0}}, "CAN"={"Device Number"=0, "SetOutput VI Ref"=variant(enum8{"Percent VBus", "Current", "Speed", "Position", "Voltage"} enum."Percent VBus"), "GetOutput VI Ref"=variant(refnum<k1> refnum), "Enable VI Ref"=variant(dbl 0.0), "Disable VI Ref"=variant(enum8{"Percent VBus", "Speed", "Position", "Slave", "Unchanged / Invalid", "Voltage Compensation", "Current", "Motion Profile"} enum."Percent VBus"), "Data"=variant}, "Invert"=FALSE}, "error out"={"status"=FALSE, "code"=0, "source"=""}}  # Left_Shooter
  w132 = T45 {"RobotDriveDevRef"={"DevStatus"={"status"=FALSE, "code"=0, "source"=""}, "Motors[]"=[], "Square Inputs"=FALSE, "Max Output"=0.0}, "error out"={"status"=FALSE, "code"=0, "source"=""}}  # Drive_Motor
  n1 = call <vilib>:"WPI_AnalogChannelRefNum Registry Get.vi"("refnum name"="Turret_Pot") -> ("error out"=w72:errorcluster, "AIDeviceRef"=w73:T15)  [unwired: 9 in]
  n2 = call <vilib>:"WPI_AnalogChannelRefNum Registry Get.vi"("refnum name"="Gear_Rail_Pot") -> ("error out"=w74:errorcluster, "AIDeviceRef"=w75:T15)  [unwired: 9 in]
  n3 = call "Ultrasonic_Ref_Get.vi"("refnum name"="Gear_Peg_Ultrasonic") -> ("error out"=w67:errorcluster, "SonarMB1010DigitalDevRef"=w68:T17)  [unwired: 1 in]
  n4 = call <vilib>:"WPI_SolenoidRefNum Registry Get.vi"("refnum name"="Gear_Chute") -> ("error out"=w42:errorcluster, "SolenoidDevRef"=w43:T26)  [unwired: 9 in]
  n5 = call <vilib>:"WPI_RobotDriveRefNum Registry Get.vi"("refnum name"="Drive_Motor") -> ("error out"=w133:errorcluster, "RobotDriveDevRef"=w134:T1)  [unwired: 9 in]
  n6 = call <vilib>:"WPI_MotorControlRefNum Registry Get.vi"("refnum name"="Left_Shooter") -> ("error out"=w122:errorcluster, "MotorControlDevRef"=w123:T2)  [unwired: 9 in]
  n7 = call <vilib>:"WPI_MotorControlRefNum Registry Get.vi"("refnum name"="Shooter_Feeder_Motor") -> ("error out"=w120:errorcluster, "MotorControlDevRef"=w121:T2)  [unwired: 9 in]
  n8 = call <vilib>:"WPI_MotorControlRefNum Registry Get.vi"("refnum name"="Intake_Motor_1") -> ("error out"=w118:errorcluster, "MotorControlDevRef"=w119:T2)  [unwired: 9 in]
  n9 = call <vilib>:"WPI_MotorControlRefNum Registry Get.vi"("refnum name"="Gear_Gate_Motor") -> ("error out"=w102:errorcluster, "MotorControlDevRef"=w101:T2)  [unwired: 9 in]
  n10 = call <vilib>:"WPI_MotorControlRefNum Registry Get.vi"("refnum name"="Climber_Motor") -> ("error out"=w85:errorcluster, "MotorControlDevRef"=w86:T2)  [unwired: 9 in]
  n11 = call "PixyCam_Refnum_Registry_Get.vi"("refnum name"="PixyCam") -> ("error out"=w13:errorcluster, "PixyCamDevRef Out"=w14:T6)  [unwired: 5 in]
  n12 = call "ADI_IMU_ADIS16448_RefNum Registry Get.vi"("refnum name"="Imu") -> ("error out"=w113:errorcluster, "ADI IMU Interrupt DevRef"=w114:T11)  [unwired: 9 in]
  n13 = call <vilib>:"WPI_AnalogChannelRefNum Registry Get.vi"("refnum name"="Gear_Gate_Pot") -> ("error out"=w76:errorcluster, "AIDeviceRef"=w77:T15)  [unwired: 9 in]
  n14 = call <vilib>:"WPI_DigitalInputRefNum Registry Get.vi"("refnum name"="Gear_Beambreak") -> ("error out"=w61:errorcluster, "DigitalInputDevRef"=w62:T23)  [unwired: 9 in]
  n15 = call <vilib>:"WPI_CompressorRefNum Registry Get.vi"("refnum name"="Compressor") -> ("error out"=w107:errorcluster, "CompressorDevRef"=w108:T25)  [unwired: 9 in]
  n16 = call <vilib>:"WPI_SolenoidRefNum Registry Get.vi"("refnum name"="Gear_Pusher") -> ("error out"=w90:errorcluster, "SolenoidDevRef"=w91:T26)  [unwired: 9 in]
  n17 = call <vilib>:"WPI_SolenoidRefNum Registry Get.vi"("refnum name"="Shifters") -> ("error out"=w98:errorcluster, "SolenoidDevRef"=w97:T26)  [unwired: 9 in]
  n18 = call <vilib>:"WPI_EncoderRefNum Registry Get.vi"("refnum name"="Shooter_Encoder") -> ("error out"=w63:errorcluster, "EncoderDevRef"=w64:T20)  [unwired: 9 in]
  n19 = call <vilib>:"WPI_DigitalInputRefNum Registry Get.vi"("refnum name"="Ball_Beambreak") -> ("error out"=w36:errorcluster, "DigitalInputDevRef"=w37:T23)  [unwired: 9 in]
  n20 = call <vilib>:"WPI_DigitalInputRefNum Registry Get.vi"("refnum name"="Gear_Orientation_Beambreak") -> ("error out"=w7:errorcluster, "DigitalInputDevRef"=w8:T23)  [unwired: 9 in]
  n21 = call <vilib>:"WPI_MotorControlRefNum Registry Get.vi"("refnum name"="Left_Turret") -> ("error out"=w80:errorcluster, "MotorControlDevRef"=w81:T2)  [unwired: 9 in]
  n22 = call <vilib>:"WPI_EncoderRefNum Registry Get.vi"("refnum name"="Drive_Encoder") -> ("error out"=w65:errorcluster, "EncoderDevRef"=w66:T20)  [unwired: 9 in]
  n23 = call <vilib>:"WPI_MotorControlRefNum Registry Get.vi"("refnum name"="Right_Shooter") -> ("error out"=w31:errorcluster, "MotorControlDevRef"=w32:T2)  [unwired: 9 in]
  n24 = call <vilib>:"WPI_MotorControlRefNum Registry Get.vi"("refnum name"="Gear_Rail_Motor") -> ("error out"=w20:errorcluster, "MotorControlDevRef"=w21:T2)  [unwired: 9 in]
  n25 = Bundle(cluster=w4, "DigitalInputDevRef"=w8, "error out"=w7) -> (w5:T31)
  n26 = Bundle(cluster=w54, "DigitalInputDevRef"=w62, "error out"=w61) -> (w57:T31)
  n27 = Bundle(cluster=w55, "EncoderDevRef"=w64, "error out"=w63) -> (w58:T42)
  n28 = Bundle(cluster=w38, "DigitalInputDevRef"=w37, "error out"=w36) -> (w34:T31)
  n29 = Bundle(cluster=w84, "MotorControlDevRef"=w86, "error out"=w85) -> (w83:T36)
  n30 = Bundle(cluster=w78, "MotorControlDevRef"=w81, "error out"=w80) -> (w79:T36)
  n31 = Bundle(cluster=w56, "EncoderDevRef"=w66, "error out"=w65) -> (w59:T42)
  n32 = Bundle(cluster=w12, "PixyCamDevRef Out"=w14, "error out"=w13) -> (w11:T34)
  n33 = Bundle(cluster=w23, "AIDeviceRef"=w77, "error out"=w76) -> (w71:T38)
  n34 = Bundle(cluster=w24, "AIDeviceRef"=w75, "error out"=w74) -> (w70:T38)
  n35 = Bundle(cluster=w25, "AIDeviceRef"=w73, "error out"=w72) -> (w69:T38)
  n36 = Bundle(cluster=w10, "SonarMB1010DigitalDevRef"=w68, "error out"=w67) -> (w60:T33)
  n37 = Bundle(cluster=w30, "MotorControlDevRef"=w32, "error out"=w31) -> (w29:T36)
  n38 = Bundle(cluster=w132, "RobotDriveDevRef"=w134, "error out"=w133) -> (w131:T45)
  n39 = Bundle(cluster=w128, "MotorControlDevRef"=w123, "error out"=w122) -> (w130:T36)
  n40 = Bundle(cluster=w127, "MotorControlDevRef"=w121, "error out"=w120) -> (w129:T36)
  n41 = Bundle(cluster=w117, "MotorControlDevRef"=w119, "error out"=w118) -> (w116:T36)
  n42 = Bundle(cluster=w100, "MotorControlDevRef"=w101, "error out"=w102) -> (w99:T36)
  n43 = Bundle(cluster=w88, "ADI IMU Interrupt DevRef"=w114, "error out"=w113) -> (w112:T43)
  n44 = Bundle(cluster=w106, "CompressorDevRef"=w108, "error out"=w107) -> (w105:T44)
  n45 = Bundle(cluster=w93, "SolenoidDevRef"=w91, "error out"=w90) -> (w89:T40)
  n46 = Bundle(cluster=w95, "SolenoidDevRef"=w97, "error out"=w98) -> (w94:T40)
  n47 = Bundle(cluster=w41, "SolenoidDevRef"=w43, "error out"=w42) -> (w40:T40)
  n48 = Bundle(cluster=w17, "MotorControlDevRef"=w21, "error out"=w20) -> (w18:T36)
  n49 = Bundle(cluster=w53, "Drive_Encoder"=w59, "Shooter_Encoder"=w58) -> (w46:T41)
  n50 = Bundle(cluster=w3, "Gear_Beambreak"=w57, "Ball_Beambreak"=w34, "Gear_Orientation_Beambreak"=w5) -> (w45:T30)
  n51 = Bundle(cluster=w22, "Gear_Gate_Pot"=w71, "Gear_Rail_Pot"=w70, "Turret_Pot"=w69) -> (w48:T37)
  n52 = Bundle(cluster=w9, "Gear_Peg_Ultrasonic"=w60) -> (w47:T32)
  n53 = Bundle(cluster=w16, "Drive_Motor"=w131, "Shooter_Motor"=w130, "Shooter_Feeder_Motor"=w129, "Intake_Motor_1"=w116, "Gear_Gate_Motor"=w99, "Climber_Motor"=w83, "Shooter_Turret_Motor"=w79, "Top_Shooter_Feeder_Motor"=w29, "Gear_Rail_Motor"=w18) -> (w111:T35)
  n54 = Bundle(cluster=w2, "PixyCam"=w11, "IMU"=w112, "Pots"=w48, "Ultrasonics"=w47, "Encoders"=w46, "DIOs"=w45) -> (w110:T29)
  n55 = Bundle(cluster=w39, "Compressor"=w105, "Gear_Pusher"=w89, "Shifters"=w94, "Gear_Chute"=w40) -> (w104:T39)
  n56 = Bundle("Motors"=w111, "Sensors"=w110, "Pneumatics"=w104) -> (→"Refnums":T28)  [unwired: 1 in]
